vi "Do bead tracking.vi"(4 "Progress notf":refnum<notifier>, 6 "Abort notf":refnum<notifier>, 8 "error in (no error)":errorcluster, 9 "Bead tracking settings":T2, 10 "Template":T3, 11 "Directory":path) -> (0 "error out":errorcluster, 3 "Results":T1[](array[typedef]) {"Raw matches"."Bounding Box"."y" format="%.2f"; "Raw matches"."Bounding Box"."x" format="%.2f"; "Raw matches"."Position"."y" format="%.2f"; "Raw matches"."Position"."x" format="%.2f"; "Raw matches"."Score" format="%.2f"; "Raw matches"."Scale" format="%.2f"; "Raw matches"."Angle" format="%.2f"})   [LabVIEW 2011]
uses:
  <vilib>/vision/Image Controls.llb/IMAQ Image.ctl
  Bead tracking settings.ctl
  Worker result.ctl
  Worker data.ctl
  COSYLib/COSYLib.lvlib
panel:
  out "Time taken per image (ms)":dbl caption="...per image" format="%#.2g ms"
  out "Time taken (s)":dbl caption="Time taken" format="%#_2f s"
  in  "# workers":u8=1 min=1 max=100
  in  "Override # workers":bool
  # "MANUAL CONTROLS"
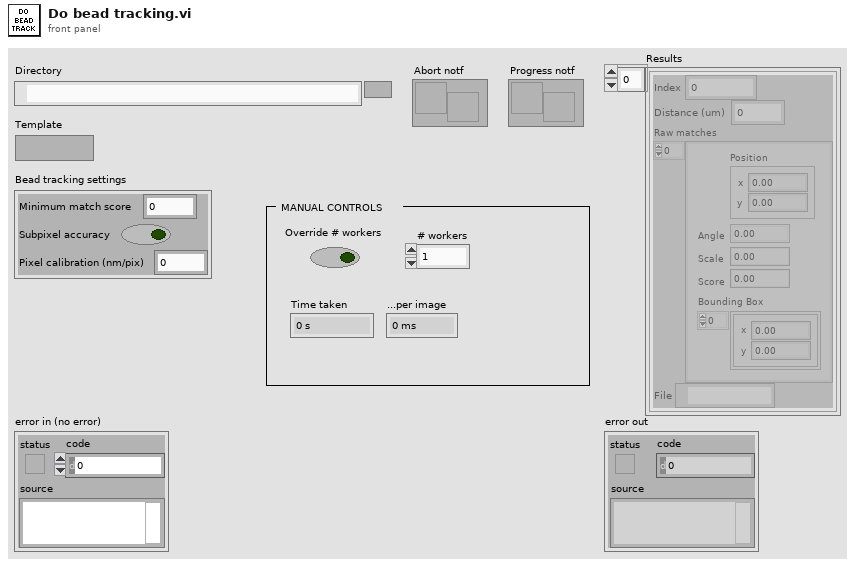
[diagram p1: front panel]
types:
  T1 = typedef "Worker result.ctl" = cluster{"Index":u32, "Distance (um)":dbl, "Raw matches":cluster{"Position":cluster{"x":sgl, "y":sgl}, "Angle":sgl, "Scale":sgl, "Score":sgl, "Bounding Box":cluster{"x":sgl, "y":sgl}[]}[], "File":path}
  T2 = typedef "Bead tracking settings.ctl" = cluster{"Minimum match score":sgl, "Subpixel accuracy":bool, "Pixel calibration (nm/pix)":dbl}
  T3 = typedef "IMAQ Image.ctl" = refnum<image>
  T4 = typedef "Worker data.ctl" = cluster{"Index":u32, "File":path}
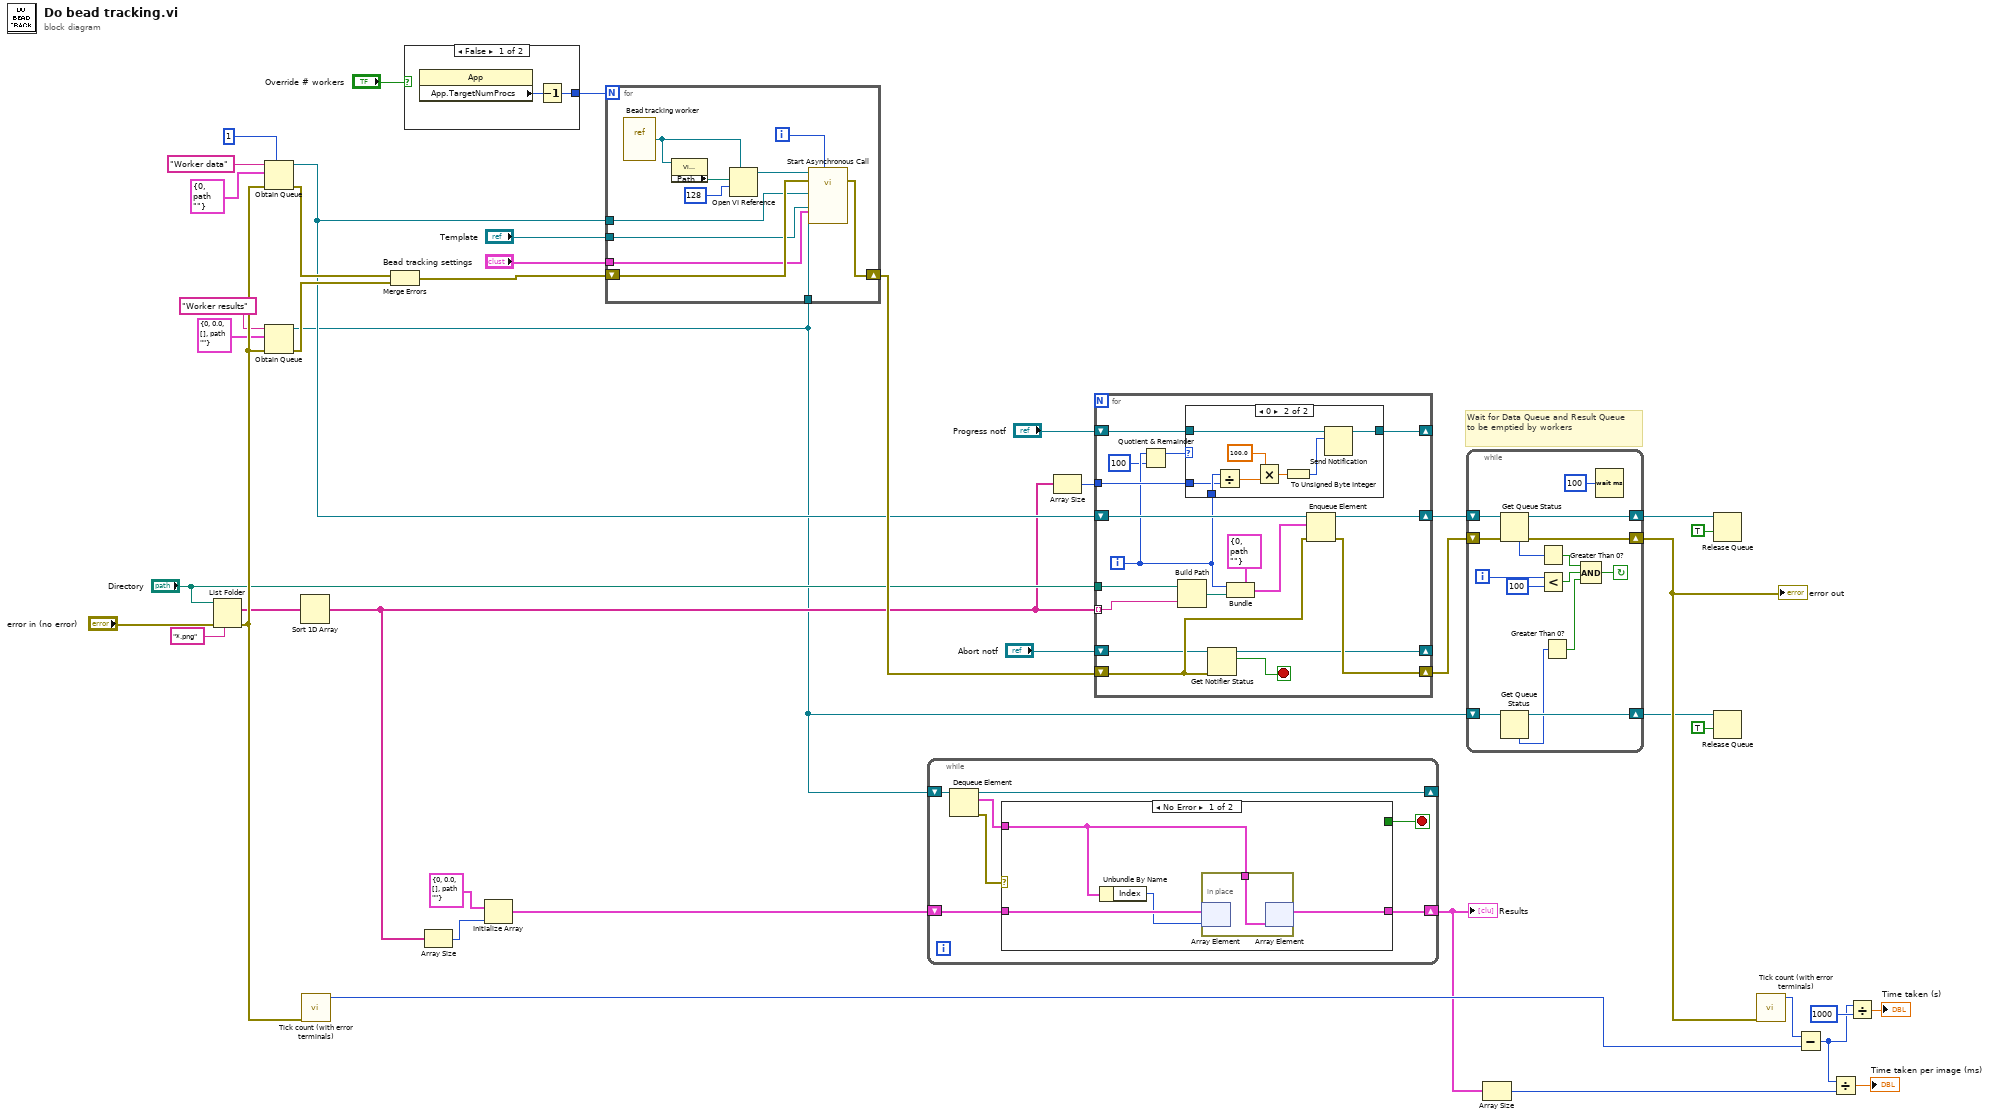
[diagram p0: block diagram]
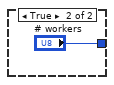
[diagram p2: hidden frame]
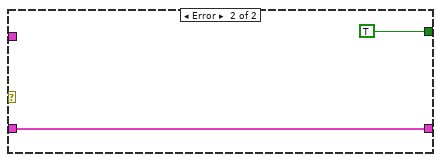
[diagram p3: hidden frame]
diagram:
  # "Wait for Data Queue and Result Queue to be emptied by workers"
  n1 = List Folder(path="Directory", pattern="*.png", error in="error in (no error)") -> (filenames=w17:string[], error out=w36:errorcluster)  [unwired: 1 in, 2 out]
  n2 = Obtain Queue(max queue size (-1, unlimited)=1, name (unnamed)="Worker data", element data type=T4 {"Index"=0, "File"=path ""} ("Worker data"), error in (no error)=w36) -> (queue out=w27:refnum<queue>, error out=w42:errorcluster)  [unwired: 1 in, 1 out]
  n3 = Obtain Queue(name (unnamed)="Worker results", element data type=T1 {"Index"=0, "Distance (um)"=0.0, "Raw matches"=[], "File"=path ""} ("Worker result"), error in (no error)=w36) -> (queue out=w13:refnum<queue>, error out=w37:errorcluster)  [unwired: 2 in, 1 out]
  n4 = Sort 1D Array(array=w17) -> (sorted array=w16:string[])
  n5 = call "Tick count (with error terminals).vi"("error in (no error)"=w36) -> ("millisecond timer value"=w7:u32)  [unwired: 9 in, 1 out]
  n6 = Merge Errors(w42, w37) -> (w38:errorcluster)
  n7 = case shown="False" "Override # workers" {
    tunnel: [w43 "# workers"] -> w34
    frame False {
      n8 = property class="App"() -> ("App.TargetNumProcs"=w44:i32)  [unwired: 2 in, 2 out]
      n9 = Decrement(x=w44) -> (x-1=w43:i32)
    }
    frame True {
    }
  }
  n10 = Array Size(array=w16) -> (size(s)=w15:i32)
  n11 = Initialize Array(T1 {"Index"=0, "Distance (um)"=0.0, "Raw matches"=[], "File"=path ""} ("Worker result"), w15) -> (w14:T1[])
  n12 = for {
    N: w34 -> [_]
    tunnel: "Template" -> [w50]
    tunnel: "Bead tracking settings" -> [w49]
    tunnel: w27 -> [w48]
    shift-right: [w56] -> w41
    shift-left: w38 -> [w55]
    tunnel: w13 -> [w46]
    i -> [w47]
    n13 = vi-ref "Bead tracking worker.vi"() -> (w53:refnum<vi>)
    n14 = property class="VI (strict)"(reference=w53) -> ("Path"=w54:path)  [unwired: 1 in, 2 out]
    n15 = Open VI Reference(type specifier VI Refnum (for type only)=w53, vi path=w54, options=128) -> (vi reference=w51:refnum<vi>)  [unwired: 3 in, 1 out]
    n16 = call-by-ref "Start Asynchronous Call"(reference=w51, error in=w55, "Bead tracking settings"=w49, "Worker index"=w47, "Template"=w50, "Result queue"=w46, "Data queue"=w48) -> (error out=w56:errorcluster)  [unwired: 7 in, 1 out]
  }
  n17 = while {
    shift-right: [w61] -> _
    shift-left: w13 -> [w62]
    shift-right: [w57] -> w6
    shift-left: w14 -> [w58]
    stop <- w59 stop-if-true
    n18 = Dequeue Element(queue=w62) -> (queue out=w61:refnum<queue>, element=w60:T1, error out=w63:errorcluster)  [unwired: 2 in, 1 out]
    n19 = case shown="No Error" w63 {
      tunnel: w60 -> [w65 _]
      tunnel: [_ TRUE] -> w59
      tunnel: w58 -> [w67 w69]
      tunnel: [w66 w69] -> w57
      frame No Error {
        n20 = Unbundle By Name(w65) -> ("Index"=w64:u32)
        n21 = in-place {
          in-place-border: w65 -> [w68]
          n22 = in-place-array #1(w67, w64) -> ()  [unwired: 1 out]
          n23 = in-place-array #1(w68) -> (w66:T1[])  [unwired: 1 out]
        }
      }
      frame Error {
      }
    }
  }
  "Results" <- w6
  n24 = Array Size(array=w16) -> (size(s)=w22:i32)
  n25 = for {
    tunnel: w16 -> [w83] mode=indexing
    shift-right: [w85] -> w21
    shift-left: w27 -> [w86]
    tunnel: "Directory" -> [w84]
    shift-right: [w78] -> _
    shift-left: "Abort notf" -> [w79]
    shift-right: [w74] -> _
    shift-left: "Progress notf" -> [w75]
    tunnel: w22 -> [w76]
    shift-right: [w88] -> w40
    shift-left: w41 -> [w87]
    i -> [w73]
    stop <- w77 stop-if-true
    n26 = Quotient & Remainder(x=w73, y=100) -> (x-y*floor(x/y)=w71:i32)  [unwired: 1 out]
    n27 = Build Path(base path=w84, name or relative path=w83) -> (appended path=w82:path)
    n28 = case shown="0" w71 {
      tunnel: w73 -> [_ w97]
      tunnel: w76 -> [_ w96]
      tunnel: w75 -> [w89 w91]
      tunnel: [w89 w90] -> w74
      frame Default {
      }
      frame 0 {
        n29 = Divide(x=w97, y=w96) -> (x/y=w95:dbl)
        n30 = Multiply(x=100.0, y=w95) -> (x*y=w93:dbl)
        n31 = To Unsigned Byte Integer(number=w93) -> (unsigned 8bit integer=w92:u8)
        n32 = Send Notification(notification=w92, notifier=w91) -> (notifier out=w90:refnum<notifier>)  [unwired: 1 in, 1 out]
      }
    }
    n33 = Get Notifier Status(notifier=w79, error in (no error)=w87) -> (notifier out=w78:refnum<notifier>, current notification=w77:bool)  [unwired: 3 out]
    n34 = Bundle(cluster=T4 {"Index"=0, "File"=path ""} ("Worker data"), "Index"=w73, "File"=w82) -> (w80:T4)
    n35 = Enqueue Element(queue=w86, element=w80, error in (no error)=w87) -> (queue out=w85:refnum<queue>, error out=w88:errorcluster)  [unwired: 1 in, 1 out]
  }
  n36 = while {
    shift-right: [w109] -> w20
    shift-left: w21 -> [w110]
    shift-right: [w111] -> w35
    shift-left: w40 -> [w112]
    shift-right: [w100] -> w11
    shift-left: w13 -> [w101]
    i -> [w106]
    stop <- w102 continue-if-true
    n37 = Get Queue Status(queue=w110, error in (no error)=w112) -> (queue out=w109:refnum<queue>, error out=w111:errorcluster, # elements in queue=w107:i32)  [unwired: 1 in, 5 out]
    n38 = Get Queue Status(queue=w101) -> (queue out=w100:refnum<queue>, # elements in queue=w99:i32)  [unwired: 2 in, 6 out]
    n39 = Greater Than 0?(x=w107) -> (x > 0?=w104:bool)
    n40 = Less?(x=w106, y=100) -> (x < y?=w103:bool)
    n41 = Greater Than 0?(x=w99) -> (x > 0?=w98:bool)
    n42 = Compound Arithmetic op=AND(w104, w103, w98) -> (w102:bool)
    n43 = Wait (ms)(milliseconds to wait=u32 100) -> ()  [unwired: 1 out]
  }
  "error out" <- w35
  n44 = Array Size(array=w6) -> (size(s)=w5:i32)
  n45 = Release Queue(queue=w20, force destroy? (F)=TRUE) -> ()  [unwired: 1 in, 3 out]
  n46 = Release Queue(queue=w11, force destroy? (F)=TRUE) -> ()  [unwired: 1 in, 3 out]
  n47 = call "Tick count (with error terminals).vi"("error in (no error)"=w35) -> ("millisecond timer value"=w8:u32)  [unwired: 9 in, 1 out]
  n48 = Subtract(x=w8, y=w7) -> (x-y=w2:u32)
  n49 = Divide(x=w2, y=w5) -> (x/y=→"Time taken per image (ms)":dbl)
  n50 = Divide(x=w2, y=u32 1000) -> (x/y=→"Time taken (s)":dbl)
